vi "Compile And Deploy.vi"(11 "target in":refnum<class "Base Target.lvclass">) -> (3 "target out":refnum<class "Base Target.lvclass">)   [LabVIEW 2020, in "NI_TargetHelper.lvlib" / "Base Target.lvclass"]
uses:
  <vilib>/TargetSupport/NI_TargetHelper/Base Target/Base Target.lvclass
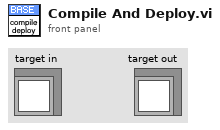
[diagram p1: front panel]
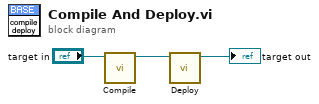
[diagram p0: block diagram]
diagram:
  n1 = call-dynamic "Compile.vi"("target in"="target in") -> ("target out"=w2:refnum<class "Base Target.lvclass">)  [unwired: 10 in]
  n2 = call-dynamic "Deploy.vi"("target in"=w2) -> ("target out"=→"target out":refnum<class "Base Target.lvclass">)  [unwired: 10 in]
